vi "Remove Frames.vi"(8 "error in (no error)":errorcluster, 9 "Frames":string[](array[string]), 10 "Action":T1, 11 "Custom Device reference in":refnum<k24>) -> (0 "error out":errorcluster, 3 "Custom Device reference out":refnum<k24>)   [LabVIEW 2023, in "J1939 System Definition API Support.lvlib"]
uses:
  J1939 System Definition API Support.lvlib
  NationalInstruments.VeriStand.SystemDefinitionAPI
  Types/Remove Frame Action.ctl
  Addon/Addon Shared/SubVIs/Constants.vi
  <vilib>/NI VeriStand/Custom Device Tools/Custom Device Utility Library/NI VeriStand - Search for All Items by GUID.vi
  <vilib>/NI VeriStand/Custom Device Tools/Custom Device Utility Library/NI VeriStand - Search for Item by Name.vi
  <vilib>/NI VeriStand/Custom Device Tools/Custom Device Utility Library/Custom Device Utility Library.lvlib
  Addon/Addon Shared/J1939 Addon Shared.lvlib
  <vilib>/NI VeriStand/Custom Device API/Custom Device API.lvlib
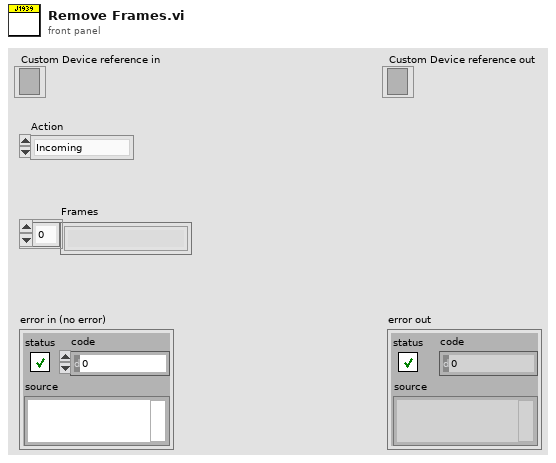
[diagram p1: front panel]
types:
  T1 = typedef "J1939 System Definition API Support.lvlib/Remove Frame Action.ctl" = enum16{"Incoming", "Outgoing Event", "Outgoing Cyclic", "Outgoing Cyclic Event"}
  T2 = typedef "Custom Device API.lvlib/Custom Device Item Ref.ctl" = u64
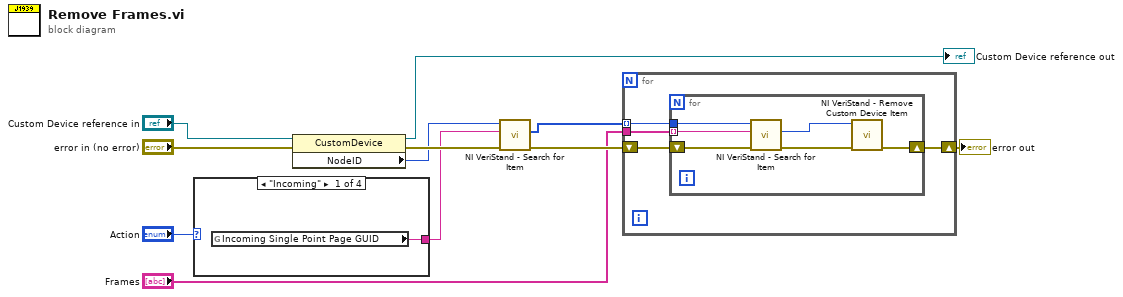
[diagram p0: block diagram]
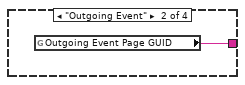
[diagram p2: hidden frame]
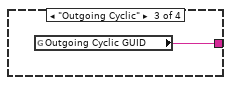
[diagram p3: hidden frame]
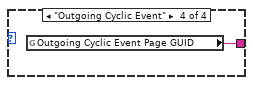
[diagram p4: hidden frame]
diagram:
  n1 = case shown="\"Incoming\"" "Action" {
    tunnel: [w12 w13 w14 w15] -> w2
    frame "Incoming" {
      n2 = global read "Constants.vi" "Incoming Single Point Page GUID"() -> (w12:string)
    }
    frame "Outgoing Event" {
      n3 = global read "Constants.vi" "Outgoing Event Page GUID"() -> (w13:string)
    }
    frame "Outgoing Cyclic" {
      n4 = global read "Constants.vi" "Outgoing Cyclic GUID"() -> (w14:string)
    }
    frame "Outgoing Cyclic Event" {
      n5 = global read "Constants.vi" "Outgoing Cyclic Event Page GUID"() -> (w15:string)
    }
  }
  n6 = property class="CustomDevice"(reference="Custom Device reference in", error in="error in (no error)") -> (reference out=→"Custom Device reference out":refnum<k24>, error out=w8:errorcluster, "NodeID"=w7:u64)
  n7 = call-poly <vilib>:"NI VeriStand - Search for Item.vi"("error in"=w8, "Item GUID"=w2, "Section Ref in"=w7) -> ("error out"=w5:errorcluster, "Item Refs"=w6:T2[])  [unwired: 5 in, 2 out]
  n8 = for {
    tunnel: w6 -> [w19] mode=indexing
    tunnel: "Frames" -> [w16]
    shift-right: [w17] -> w4
    shift-left: w5 -> [w18]
    n9 = for {
      tunnel: w19 -> [w25]
      tunnel: w16 -> [w23] mode=indexing
      shift-right: [w20] -> w17
      shift-left: w18 -> [w24]
      n10 = call-poly <vilib>:"NI VeriStand - Search for Item.vi"("error in"=w24, "Item Name"=w23, "Section Ref in"=w25) -> ("error out"=w21:errorcluster, "Item Ref"=w22:T2)  [unwired: 5 in, 2 out]
      n11 = call <vilib>:"NI VeriStand - Remove Custom Device Item.vi"("error in (no error)"=w21, "Item Ref in"=w22) -> ("error out"=w20:errorcluster)  [unwired: 8 in, 1 out]
    }
  }
  "error out" <- w4
